vi "configEstacion_toArduino_QR.vi"(8 "error in (no error)":errorcluster, 9 "LECTURA QR INPUT":T1={"COORD X"=0, "COORD  Y"=0, "NºASICS"=1, "SELECCIÓN DE BANDEJA"=enum."BANDEJA ENTRADA", "CONTEO QR"=0}, 10 "Configuracion Estación":T2={"Coordenadas_estacion"={"Coord.Bandeja entrada"={"Coord. X0 entrada"=0, "Coord. Y0 entrada "=0, "Altura Z entrada"=0}, "Coord.Bandeja OK"={"Coord. X0 OK"=0, "Coord. Y0 OK"=0, "Altura Z OK"=0}, "Coord.Bandeja entrada FAIL"={"Coord. X0 FAIL"=0, "Coord. Y0 FAIL"=0, "Altura Z FAIL"=0}, "Coord. Socket"={"Coord. X socket"=0, "Coord. Y socket"=0, "Altura Z socket"=0}}, "Nombre Bandeja"="", "Datos bandeja"={"Nº de columnas "=0, "Nº de filas "=0, "largo"=0, "ancho"=0, "nombre"="nombre", "Paso X (en mm)"=0.0, "Paso Y (en mm)"=0.0, "DISTANCIA SUELO A CHIP  "=0.0, "Nº de celdas totales"=0, "Distancia chips bandejas contiguas"=0.0}}, 11 "VISA resource name":refnum<visa-resource-name>) -> (0 "error IO":errorcluster, 2 "datos leídos":string, 3 "trama datos enviada":string)   [LabVIEW 2019]
uses:
  LVPROJ_CONFIG_ESTACION/Type_defs/Coordenadas_estacion.ctl
  LVPROJ_CREAR BANDEJAS/Type_defs/Data_Bandeja.ctl
  TYPE'S DEF/INPUT LECTURA_QR.ctl
  <vilib>/Utility/error.llb/Error Cluster From Error Code.vi
  <vilib>/ErrorRing/Error Ring.xnode
  SHARED VI'S/SHARED VI'S.lvlib
panel:
  out "return count":u32
  # "CELDA DE COMIENZO"
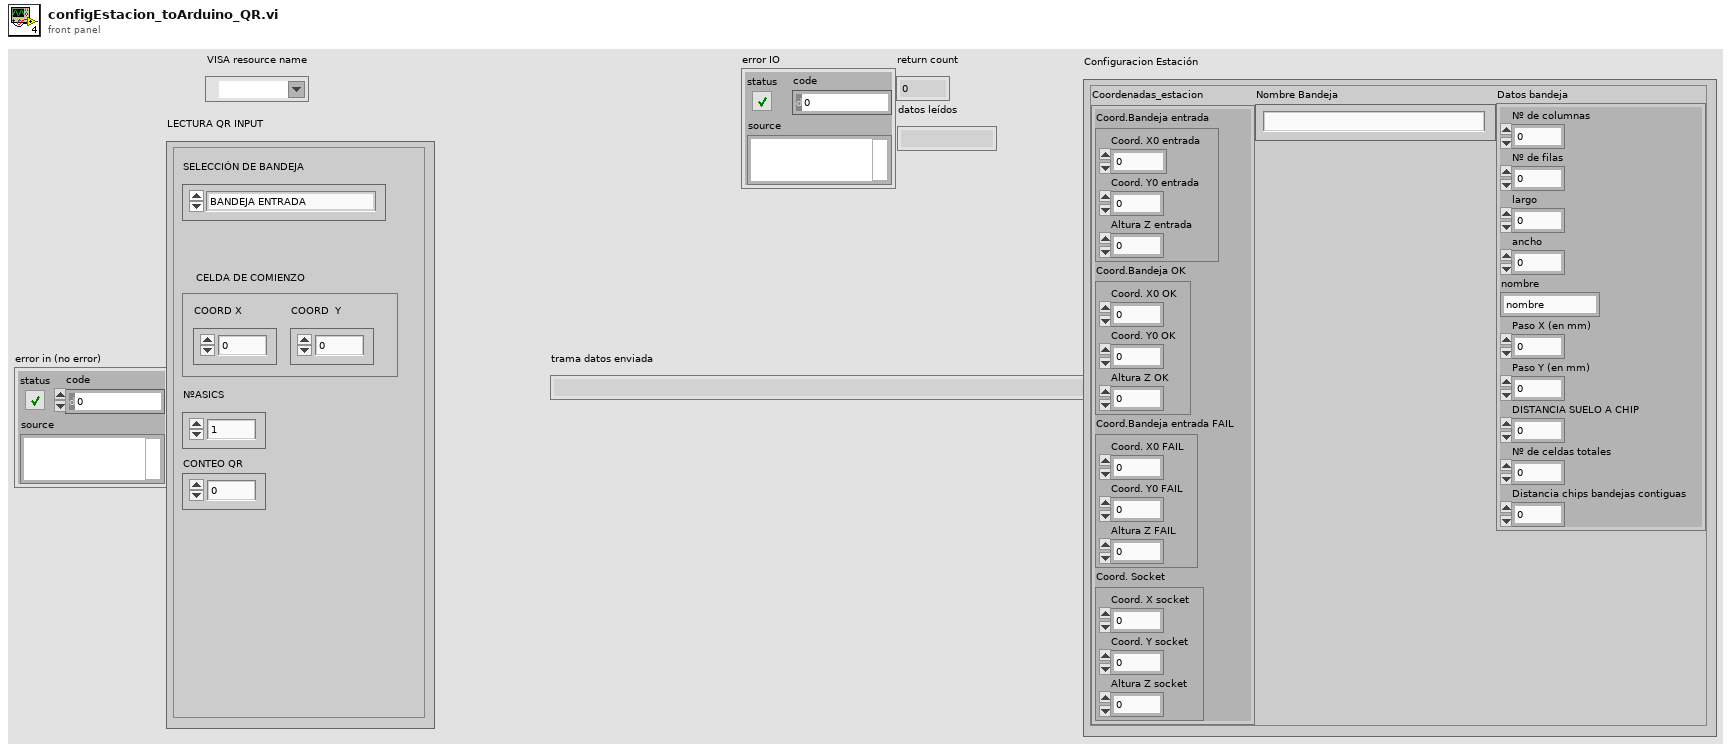
[diagram p1: front panel]
types:
  T1 = typedef "INPUT LECTURA_QR.ctl" = cluster{"COORD X":u16, "COORD  Y":u16, "NºASICS":u32, "SELECCIÓN DE BANDEJA":enum16{"BANDEJA ENTRADA", "BANDEJA OK", "BANDEJA NOK"}, "CONTEO QR":u32}
  T2 = typedef "Configuracion_estación.ctl" = cluster{"Coordenadas_estacion":T3, "Nombre Bandeja":string, "Datos bandeja":T4}
  T3 = typedef "Coordenadas_estacion.ctl" = cluster{"Coord.Bandeja entrada":cluster{"Coord. X0 entrada":u32, "Coord. Y0 entrada ":u32, "Altura Z entrada":u32}, "Coord.Bandeja OK":cluster{"Coord. X0 OK":u32, "Coord. Y0 OK":u32, "Altura Z OK":u32}, "Coord.Bandeja entrada FAIL":cluster{"Coord. X0 FAIL":u32, "Coord. Y0 FAIL":u32, "Altura Z FAIL":u32}, "Coord. Socket":cluster{"Coord. X socket":u32, "Coord. Y socket":u32, "Altura Z socket":u32}}
  T4 = typedef "Data_Bandeja.ctl" = cluster{"Nº de columnas ":u32, "Nº de filas ":u32, "largo":u32, "ancho":u32, "nombre":string, "Paso X (en mm)":dbl, "Paso Y (en mm)":dbl, "DISTANCIA SUELO A CHIP  ":dbl, "Nº de celdas totales":u16, "Distancia chips bandejas contiguas":dbl}
  T5 = enum16{"BANDEJA ENTRADA", "BANDEJA OK", "BANDEJA NOK"}
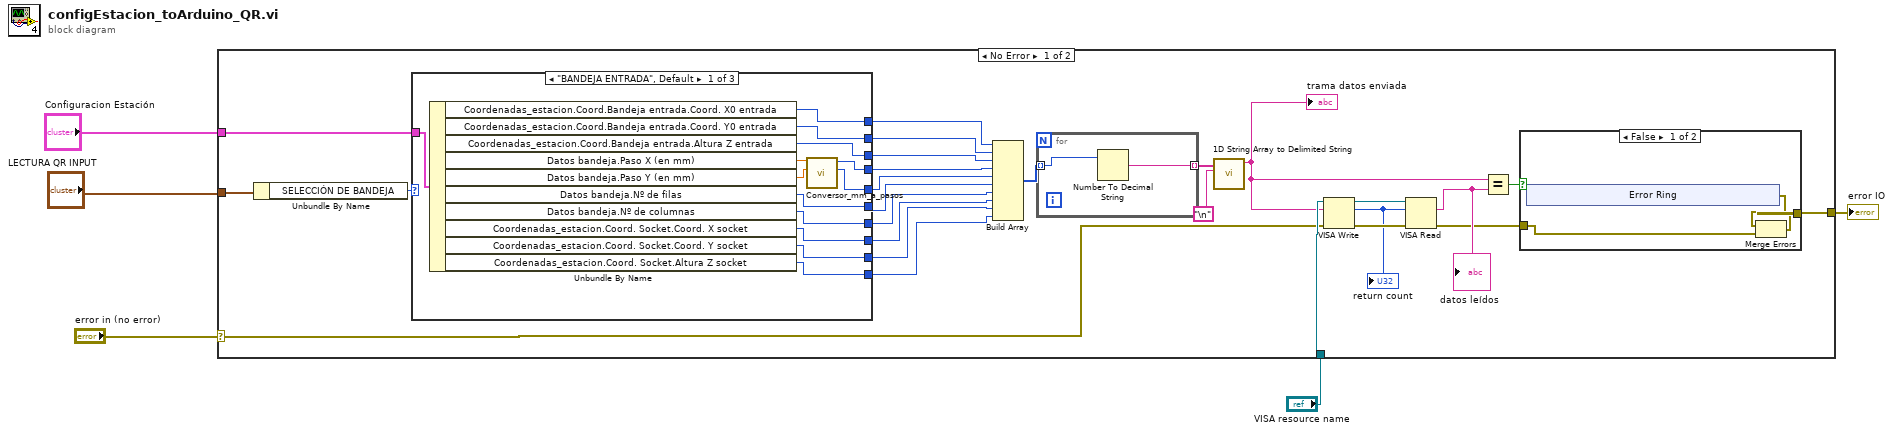
[diagram p0: block diagram]
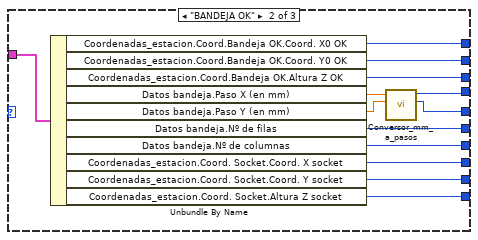
[diagram p2: hidden frame]
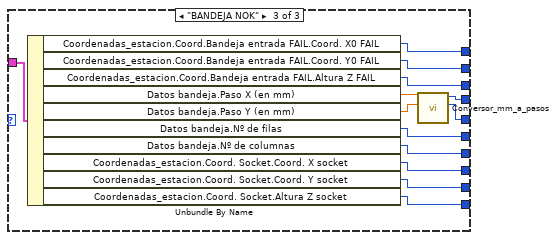
[diagram p3: hidden frame]
diagram:
  n1 = case shown="No Error" "error in (no error)" {
    selector: "error in (no error)" -> [w27 w82]
    tunnel: "Configuracion Estación" -> [w16 _]
    tunnel: "VISA resource name" -> [w28 _]
    tunnel: [w20 w82] -> w2
    tunnel: "LECTURA QR INPUT" -> [w18 _]
    frame No Error {
      n2 = Unbundle By Name(w18) -> ("SELECCIÓN DE BANDEJA"=w17:T5)
      n3 = case shown="\"BANDEJA ENTRADA\", Default" w17 {
        tunnel: w16 -> [w44 w53 w70]
        tunnel: [w43 w57 w69] -> w15
        tunnel: [w42 w56 w68] -> w14
        tunnel: [w41 w55 w67] -> w13
        tunnel: [w33 w51 w59] -> w12
        tunnel: [w32 w50 w58] -> w11
        tunnel: [w38 w54 w62] -> w10
        tunnel: [w37 w49 w63] -> w9
        tunnel: [w36 w48 w64] -> w8
        tunnel: [w35 w47 w65] -> w7
        tunnel: [w34 w46 w66] -> w6
        frame "BANDEJA ENTRADA", Default {
          n4 = Unbundle By Name(w44) -> ("Coordenadas_estacion.Coord.Bandeja entrada.Coord. X0 entrada"=w43:u32, "Coordenadas_estacion.Coord.Bandeja entrada.Coord. Y0 entrada"=w42:u32, "Coordenadas_estacion.Coord.Bandeja entrada.Altura Z entrada"=w41:u32, "Datos bandeja.Paso X (en mm)"=w40:dbl, "Datos bandeja.Paso Y (en mm)"=w39:dbl, "Datos bandeja.Nº de filas"=w38:u32, "Datos bandeja.Nº de columnas"=w37:u32, "Coordenadas_estacion.Coord. Socket.Coord. X socket"=w36:u32, "Coordenadas_estacion.Coord. Socket.Coord. Y socket"=w35:u32, "Coordenadas_estacion.Coord. Socket.Altura Z socket"=w34:u32)
          n5 = call "Conversor_mm_a_pasos.vi"("pasosY"=w39, "pasosX"=w40) -> ("PASOS EN Y"=w32:u32, "PASOS EN X"=w33:u32)  [unwired: 6 in, 2 out]
        }
        frame "BANDEJA OK" {
          n6 = Unbundle By Name(w53) -> ("Coordenadas_estacion.Coord.Bandeja OK.Coord. X0 OK"=w57:u32, "Coordenadas_estacion.Coord.Bandeja OK.Coord. Y0 OK"=w56:u32, "Coordenadas_estacion.Coord.Bandeja OK.Altura Z OK"=w55:u32, "Datos bandeja.Paso X (en mm)"=w52:dbl, "Datos bandeja.Paso Y (en mm)"=w45:dbl, "Datos bandeja.Nº de filas"=w54:u32, "Datos bandeja.Nº de columnas"=w49:u32, "Coordenadas_estacion.Coord. Socket.Coord. X socket"=w48:u32, "Coordenadas_estacion.Coord. Socket.Coord. Y socket"=w47:u32, "Coordenadas_estacion.Coord. Socket.Altura Z socket"=w46:u32)
          n7 = call "Conversor_mm_a_pasos.vi"("pasosY"=w45, "pasosX"=w52) -> ("PASOS EN Y"=w50:u32, "PASOS EN X"=w51:u32)  [unwired: 6 in, 2 out]
        }
        frame "BANDEJA NOK" {
          n8 = Unbundle By Name(w70) -> ("Coordenadas_estacion.Coord.Bandeja entrada FAIL.Coord. X0 FAIL"=w69:u32, "Coordenadas_estacion.Coord.Bandeja entrada FAIL.Coord. Y0 FAIL"=w68:u32, "Coordenadas_estacion.Coord.Bandeja entrada FAIL.Altura Z FAIL"=w67:u32, "Datos bandeja.Paso X (en mm)"=w61:dbl, "Datos bandeja.Paso Y (en mm)"=w60:dbl, "Datos bandeja.Nº de filas"=w62:u32, "Datos bandeja.Nº de columnas"=w63:u32, "Coordenadas_estacion.Coord. Socket.Coord. X socket"=w64:u32, "Coordenadas_estacion.Coord. Socket.Coord. Y socket"=w65:u32, "Coordenadas_estacion.Coord. Socket.Altura Z socket"=w66:u32)
          n9 = call "Conversor_mm_a_pasos.vi"("pasosY"=w60, "pasosX"=w61) -> ("PASOS EN Y"=w58:u32, "PASOS EN X"=w59:u32)  [unwired: 6 in, 2 out]
        }
      }
      n10 = Build Array(w15, w14, w13, w12, w11, w10, w9, w8, w7, w6) -> (w31:u32[])
      n11 = for {
        tunnel: w31 -> [w80] mode=indexing
        tunnel: [w81] -> w30 mode=indexing
        n12 = Number To Decimal String(number=w80) -> (decimal integer string=w81:string)  [unwired: 1 in]
      }
      n13 = call <vilib>:"1D String Array to Delimited String.vi"("delimiter"="\n", "string array"=w30) -> ("delimited string"=w23:string)  [unwired: 9 in]
      "trama datos enviada" <- w23
      n14 = VISA Write(VISA resource name=w28, write buffer=w23, error in (no error)=w27) -> (VISA resource name out=w25:refnum<visa-resource-name>, return count=w24:u32, error out=w26:errorcluster)
      "return count" <- w24
      n15 = VISA Read(VISA resource name=w25, byte count=w24, error in (no error)=w26) -> (read buffer=w22:string, error out=w19:errorcluster)  [unwired: 2 out]
      "datos leídos" <- w22
      n16 = Equal?(x=w23, y=w22) -> (x = y?=w21:bool)
      n17 = case shown="False" w21 {
        tunnel: [w73 w79] -> w20
        tunnel: w19 -> [w71 w79]
        frame False {
          n18 = xnode "Error Ring"() -> ("error out"=w72:errorcluster)
          n19 = Merge Errors(w72, w71) -> (w73:errorcluster)
        }
        frame True {
        }
      }
    }
    frame Error {
    }
  }
  "error IO" <- w2
